vi "modbus-conver.vi"(6 "Reg":dbl, 8 "error in (no error)":errorcluster, 9 "Scale Min range":dbl, 10 "Scale Max Range":dbl, 11 "object in":refnum<class "Modbus-Instr.lvclass">) -> (0 "error out":errorcluster, 2 "output":dbl, 3 "object out":refnum<class "Modbus-Instr.lvclass">)   [LabVIEW 2021, in "Modbus-Instr.lvclass"]
doc: "formula to convert adam modbus to real"
uses:
  Modbus-Instr.lvclass
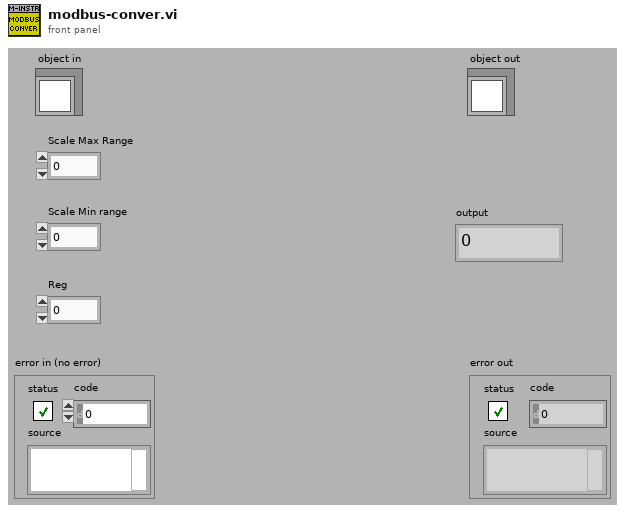
[diagram p1: front panel]
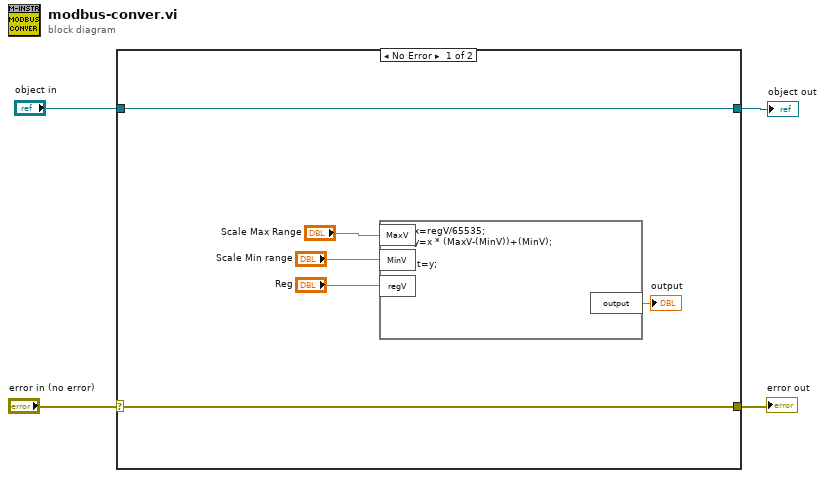
[diagram p0: block diagram]
diagram:
  n1 = case shown="No Error" "error in (no error)" {
    selector: "error in (no error)" -> [w10 w12]
    tunnel: [w10 w12] -> w3
    tunnel: [w9 w11] -> w1
    tunnel: "object in" -> [w9 w11]
    frame No Error {
      n2 = formula code="float x=regV/65535;\nfloat y=x * (MaxV-(MinV))+(MinV);\n\noutput=y;"("MaxV"="Scale Max Range", "MinV"="Scale Min range", "regV"="Reg") -> ("output"=→"output":dbl)
    }
    frame Error {
    }
  }
  "error out" <- w3
  "object out" <- w1
